vi "Get ACS version.vi"(8 "error in (no error)":errorcluster, 11 "Channel in":refnum<class "SPARC4_Channel.lvclass">) -> (0 "error out":errorcluster, 2 "ACS version":string, 3 "Channel out":refnum<class "SPARC4_Channel.lvclass">)   [LabVIEW 2018, in "SPARC4_Channel.lvclass"]
doc: "Get the ACS version"
uses:
  SPARC4_Channel.lvclass
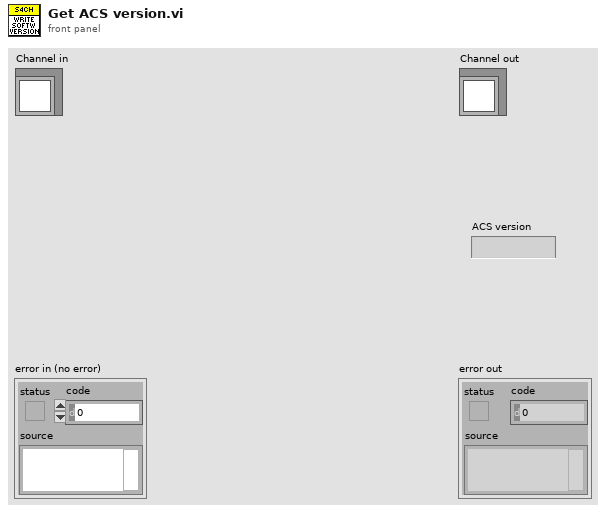
[diagram p1: front panel]
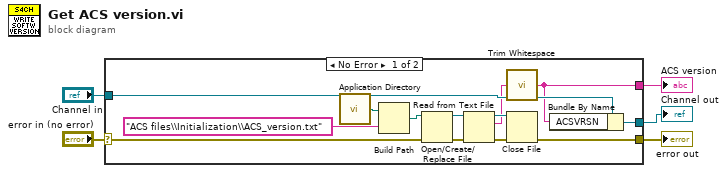
[diagram p0: block diagram]
diagram:
  n1 = case shown="No Error" "error in (no error)" {
    selector: "error in (no error)" -> [w17 w20]
    tunnel: [w18 w20] -> w4
    tunnel: [w15 w19] -> w2
    tunnel: "Channel in" -> [w16 w19]
    tunnel: [w14 _] -> w1
    frame No Error {
      n2 = call <vilib>:"Application Directory.vi"() -> ("Application Directory"=w8:path)
      n3 = Build Path(base path=w8, name or relative path="ACS files\\Initialization\\ACS_version.txt") -> (appended path=w9:path)
      n4 = Open/Create/Replace File(file path (use dialog)=w9, error in=w17) -> (refnum out=w13:refnum<file>, error out=w12:errorcluster)  [unwired: 4 in, 1 out]
      n5 = Read from Text File(file (use dialog)=w13, error in=w12) -> (refnum out=w10:refnum<file>, text=w6:string, error out=w11:errorcluster)  [unwired: 2 in, 1 out]
      n6 = call <vilib>:"Trim Whitespace.vi"("string"=w6) -> ("trimmed string"=w14:string)  [unwired: 1 in]
      n7 = Close File(refnum=w10, error in=w11) -> (error out=w18:errorcluster)  [unwired: 1 out]
      n8 = Bundle By Name(cluster=w16, "ACSVRSN"=w14) -> (w15:refnum<class "SPARC4_Channel.lvclass">)
    }
    frame Error {
    }
  }
  "error out" <- w4
  "Channel out" <- w2
  "ACS version" <- w1
